vi "Host_Model_Updating.vi"(11 "Setup Parameters and Controls":T3={"Modeling Parameters input controls"={"beam_length"=0.3525, "youngs_modulus"=209500000000.0, "torsion_spring"=0.0, "beam_height"=0.00635, "beam_width"=0.0508, "beam_density"=7900.0, "number_of_FEA_nodes"=40, "accelerometer_mass"=0.055}, "Mockbear input controls"={"Dataset"="test7", "Resample Method"=enum."Auto Resample"}, "Simulation Parameters input controls"={"Eigensolver "=enum."LEMP", "Models Forcasted"=5, "Max Roller Velocity"=3.32, "Max Roller Position Percent"=0.43, "Min Roller Position Percent"=0.155}, "Program Controls"={"Frequency KF"=TRUE, "Pinned State KF"=FALSE, "FFT Bounding"=FALSE, "Filter Constants Frequency"={"Measurement Variance"=0.4, "State Variance"=0.01, "Threshold"=1000000000.0}, "Filter Constants Position"={"Measurement Variance"=0.4, "State Variance"=0.9, "Threshold"=1000000000.0}, "Moving Window Size"=10, "Time Series buffer"=10000.0, "Record Time Series Data"=FALSE, "Record Moving Window Data"=FALSE, "Record Online Error Metrics "=TRUE, "Record Statistics"=TRUE}}) -> ()   [LabVIEW 2021]
uses:
  Model_Updating_Classes/DROPBEAR_Model_Updating/DROPBEAR_Model_Updating.lvclass
panel:
  in  "Tab Control":enum32{"Time Series", "Statistics", "Controls"}(tab)
  out "Frequency":dynamicdata(graph)
  out "Meter":dynamicdata(graph)
  out "Nodal":dynamicdata(graph)
  out "DAQ Time cost":T1
  out "FFT Time cost":T1
  out "FEA Time cost":T1
  out "FFT KF Time cost":T1
  out "Sampling Time cost":T1
  out "State KF Time cost":T1
  out "Cycle Time cost":T1
  out "StatisticsTime cost":T1
  out "Signal Quality Stats Frequency":T2
  out "Signal Quality Stats Position":T2
  out "Average Cycle Time (ms)":dbl
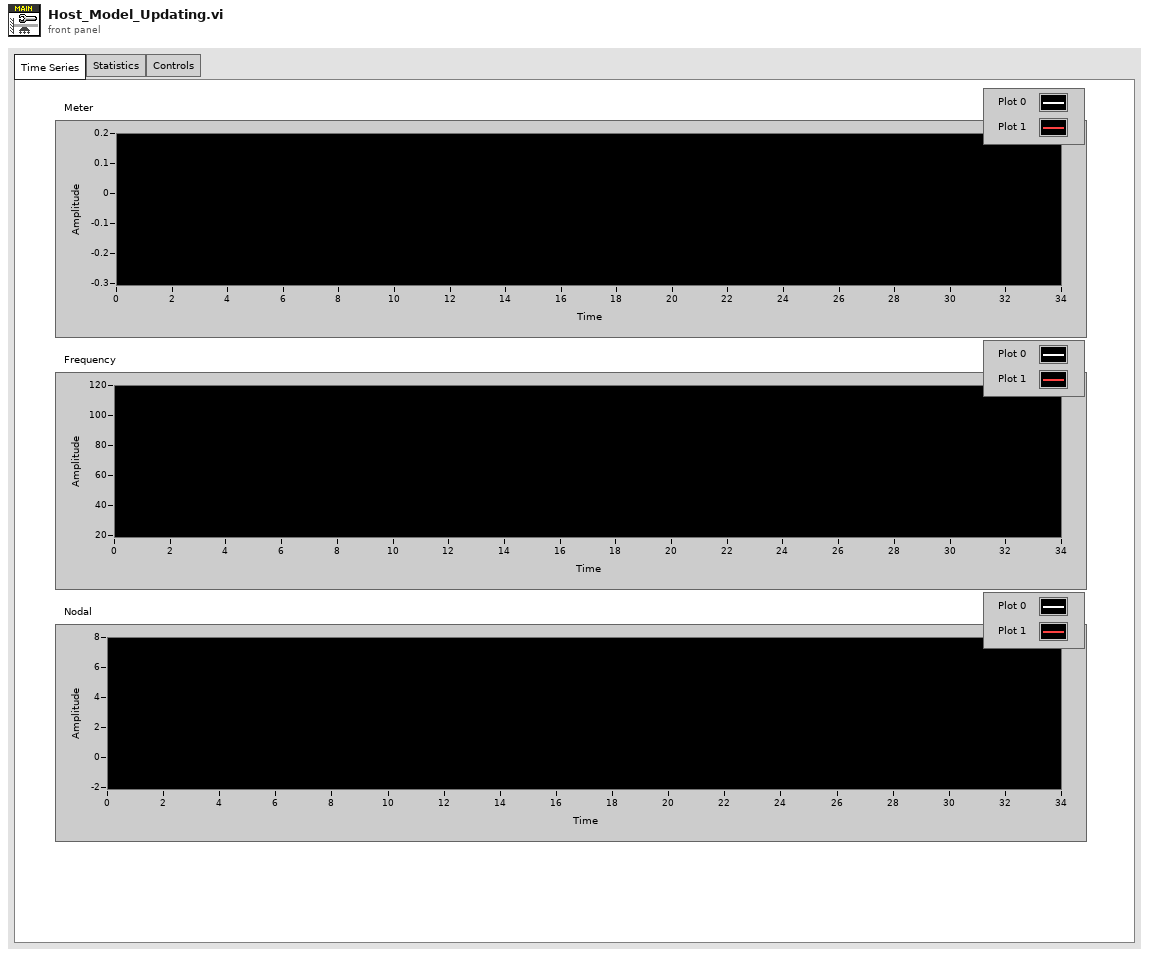
[diagram p1: front panel]
types:
  T1 = cluster{"Cumulative_mean":dbl, "Cumulative_mean_square ":dbl, "Cumulative_variance":dbl, "Max":dbl, "Min":dbl, "Number_of_samples":i32}
  T2 = cluster{"SNR":dbl, "TRAC":dbl, "Cumulative_mean":dbl, "Cumulative_mean_square ":dbl, "Cumulative_variance":dbl, "Max":dbl, "Min":dbl, "Number_of_samples":i32}
  T3 = cluster{"Modeling Parameters input controls":cluster{"beam_length":dbl, "youngs_modulus":dbl, "torsion_spring":dbl, "beam_height":dbl, "beam_width":dbl, "beam_density":dbl, "number_of_FEA_nodes":i32, "accelerometer_mass":dbl}, "Mockbear input controls":cluster{"Dataset":string, "Resample Method":enum16{"Recorded", "Auto Resample", "Custom Resample"}}, "Simulation Parameters input controls":cluster{"Eigensolver ":enum16{"LabVIEW Cholesky", "LabVIEW General", "LabVIEW Inverse", "LEMP"}, "Models Forcasted":i32, "Max Roller Velocity":dbl, "Max Roller Position Percent":dbl, "Min Roller Position Percent":dbl}, "Program Controls":cluster{"Frequency KF":bool, "Pinned State KF":bool, "FFT Bounding":bool, "Filter Constants Frequency":cluster{"Measurement Variance":dbl, "State Variance":dbl, "Threshold":dbl}, "Filter Constants Position":cluster{"Measurement Variance":dbl, "State Variance":dbl, "Threshold":dbl}, "Moving Window Size":i32, "Time Series buffer":dbl, "Record Time Series Data":bool, "Record Moving Window Data":bool, "Record Online Error Metrics ":bool, "Record Statistics":bool}}
  T4 = cluster{"Signal Quality Stats Frequency":cluster{"SNR":dbl, "TRAC":dbl, "Cumulative_mean":dbl, "Cumulative_mean_square ":dbl, "Cumulative_variance":dbl, "Max":dbl, "Min":dbl, "Number_of_samples":i32}, "Signal Quality Stats Position":cluster{"SNR":dbl, "TRAC":dbl, "Cumulative_mean":dbl, "Cumulative_mean_square ":dbl, "Cumulative_variance":dbl, "Max":dbl, "Min":dbl, "Number_of_samples":i32}}
  T5 = cluster{"DAQ Time cost":cluster{"Cumulative_mean":dbl, "Cumulative_mean_square ":dbl, "Cumulative_variance":dbl, "Max":dbl, "Min":dbl, "Number_of_samples":i32}, "FFT Time cost":cluster{"Cumulative_mean":dbl, "Cumulative_mean_square ":dbl, "Cumulative_variance":dbl, "Max":dbl, "Min":dbl, "Number_of_samples":i32}, "FFT KF Time cost":cluster{"Cumulative_mean":dbl, "Cumulative_mean_square ":dbl, "Cumulative_variance":dbl, "Max":dbl, "Min":dbl, "Number_of_samples":i32}, "Sampling Time cost":cluster{"Cumulative_mean":dbl, "Cumulative_mean_square ":dbl, "Cumulative_variance":dbl, "Max":dbl, "Min":dbl, "Number_of_samples":i32}, "FEA Time cost":cluster{"Cumulative_mean":dbl, "Cumulative_mean_square ":dbl, "Cumulative_variance":dbl, "Max":dbl, "Min":dbl, "Number_of_samples":i32}, "State KF Time cost":cluster{"Cumulative_mean":dbl, "Cumulative_mean_square ":dbl, "Cumulative_variance":dbl, "Max":dbl, "Min":dbl, "Number_of_samples":i32}, "Cycle Time cost":cluster{"Cumulative_mean":dbl, "Cumulative_mean_square ":dbl, "Cumulative_variance":dbl, "Max":dbl, "Min":dbl, "Number_of_samples":i32}, "StatisticsTime cost":cluster{"Cumulative_mean":dbl, "Cumulative_mean_square ":dbl, "Cumulative_variance":dbl, "Max":dbl, "Min":dbl, "Number_of_samples":i32}}
  T6 = cluster{"Frequency":dynamicdata, "Meters":dynamicdata, "Nodal":dynamicdata}
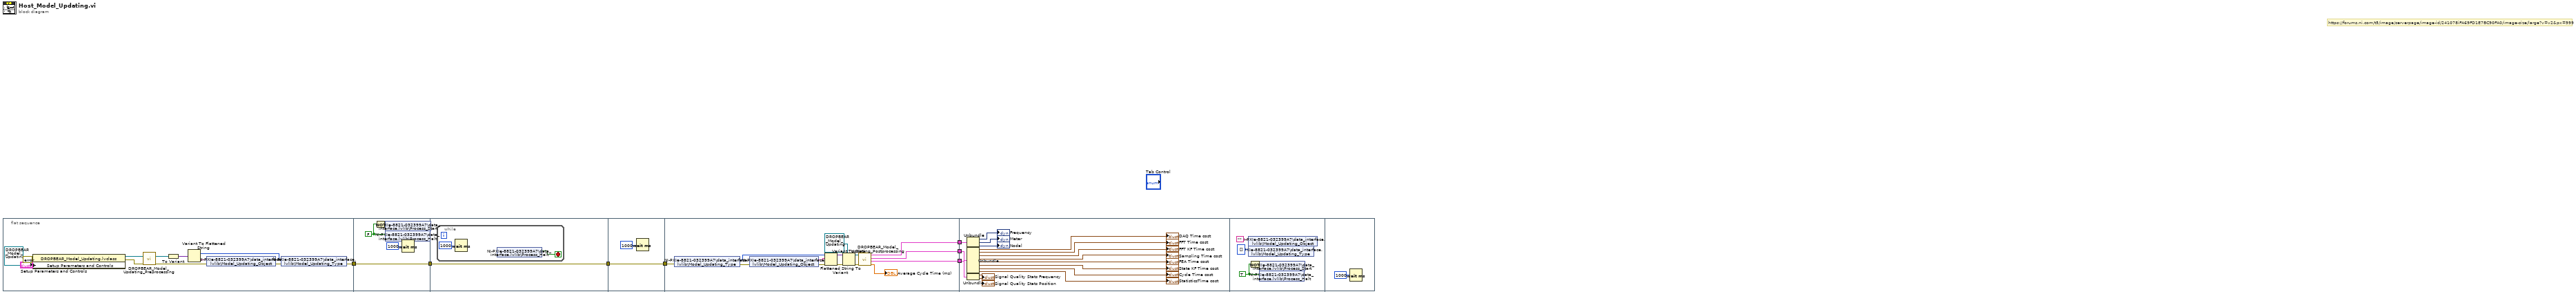
[diagram p0: block diagram]
diagram:
  # "https://forums.ni.com/t5/image/serverpage/image-id/241078iFA69FD1E7BC90FA0/image-size/large?v=v2&px=999"
  n1 = flat-sequence {
    tunnel: [w14] -> w4
    tunnel: w4 -> [w20]
    tunnel: [w20] -> w1
    tunnel: [w24] -> w3
    tunnel: w1 -> [w24]
    tunnel: w3 -> [w27]
    tunnel: [w27] -> w2
    tunnel: [w31] -> w7
    tunnel: [w30] -> w6
    tunnel: [w29] -> w5
    tunnel: w2 -> [w34]
    tunnel: w5 -> [w58]
    tunnel: w6 -> [w55]
    tunnel: w7 -> [w46]
    frame #0 {
      n2 = property class="DROPBEAR_Model_Updating.lvclass"(reference=refnum<class "DROPBEAR_Model_Updating.lvclass"> refnum ("DROPBEAR_Model_Updating.lvclass"), error in=errorcluster {"status"=FALSE, "code"=0, "source"=""} ("error in (no error)"), "Setup Parameters and Controls"="Setup Parameters and Controls") -> (reference out=w13:refnum<class "DROPBEAR_Model_Updating.lvclass">, error out=w9:errorcluster)
      n3 = call-dynamic "DROPBEAR_Model_Updating_Preprocessing.vi"("error in (no error)"=w9, "DROPBEAR_Model_Updating in"=w13) -> ("error out"=w18:errorcluster, "DROPBEAR_Model_Updating out"=w19:refnum<class "DROPBEAR_Model_Updating.lvclass">)  [unwired: 8 in]
      n4 = To Variant(anything=w19) -> (Variant=w17:variant)
      n5 = Variant To Flattened String(Variant=w17) -> (data string=w16:string, 1:w8:i16[])
      n6 = shared-variable "NI-PXIe-8821-032399A7\\data_interface.lvlib\\Model_Updating_Object"(w16, error in=w18) -> (error out=w15:errorcluster)
      n7 = shared-variable "NI-PXIe-8821-032399A7\\data_interface.lvlib\\Model_Updating_Type"(w8, error in=w15) -> (error out=w14:errorcluster)
    }
    frame #1 {
      w21 = FALSE ("Process_Halt")
      n8 = Not(x=w21) -> (.not. x?=w22:bool)
      n9 = shared-variable "NI-PXIe-8821-032399A7\\data_interface.lvlib\\Process_Start"(w22) -> ()  [unwired: 1 in, 1 out]
      n10 = shared-variable "NI-PXIe-8821-032399A7\\data_interface.lvlib\\Process_Halt"(w21) -> ()  [unwired: 1 in, 1 out]
      n11 = Wait (ms)(milliseconds to wait=u32 1000) -> ()  [unwired: 1 out]
    }
    frame #2 {
      n12 = while {
        stop <- w26 stop-if-true
        n13 = Wait (ms)(milliseconds to wait=u32 1000) -> ()  [unwired: 1 out]
        n14 = shared-variable "NI-PXIe-8821-032399A7\\data_interface.lvlib\\Process_Halt"() -> (w26:bool)  [unwired: 1 in, 1 out]
      }
    }
    frame #3 {
      n15 = Wait (ms)(milliseconds to wait=u32 1000) -> ()  [unwired: 1 out]
    }
    frame #4 {
      n16 = shared-variable "NI-PXIe-8821-032399A7\\data_interface.lvlib\\Model_Updating_Type"(error in=w34) -> (w38:i16[], error out=w41:errorcluster)
      n17 = shared-variable "NI-PXIe-8821-032399A7\\data_interface.lvlib\\Model_Updating_Object"(error in=w41) -> (w39:string, error out=w40:errorcluster)
      n18 = Flattened String To Variant(4:w40, 6:w39, 7:w38) -> (0:w35:errorcluster, 3:w36:variant)
      n19 = Variant To Data(error in=w35, type=refnum<class "DROPBEAR_Model_Updating.lvclass"> refnum ("DROPBEAR_Model_Updating.lvclass"), Variant=w36) -> (data=w33:refnum<class "DROPBEAR_Model_Updating.lvclass">, error out=w32:errorcluster)
      n20 = call "DROPBEAR_Model_Updating_Postprocessing.vi"("error in (no error)"=w32, "DROPBEAR_Model_Updating in"=w33) -> ("Cycle time (ms)"=→"Average Cycle Time (ms)":dbl, "Signal Quality"=w29:T4, "Timing stats"=w30:T5, "Plots"=w31:T6)  [unwired: 6 in]
    }
    frame #5 {
      n21 = Unbundle(w46) -> ("Frequency"=→"Frequency":dynamicdata, "Meters"=→"Meter":dynamicdata, "Nodal"=→"Nodal":dynamicdata)
      n22 = Unbundle(w55) -> ("DAQ Time cost"=→"DAQ Time cost":T1, "FFT Time cost"=→"FFT Time cost":T1, "FFT KF Time cost"=→"FFT KF Time cost":T1, "Sampling Time cost"=→"Sampling Time cost":T1, "FEA Time cost"=→"FEA Time cost":T1, "State KF Time cost"=→"State KF Time cost":T1, "Cycle Time cost"=→"Cycle Time cost":T1, "StatisticsTime cost"=→"StatisticsTime cost":T1)
      n23 = Unbundle(w58) -> ("Signal Quality Stats Frequency"=→"Signal Quality Stats Frequency":T2, "Signal Quality Stats Position"=→"Signal Quality Stats Position":T2)
    }
    frame #6 {
      w60 = TRUE ("Process_Halt")
      n24 = shared-variable "NI-PXIe-8821-032399A7\\data_interface.lvlib\\Model_Updating_Object"("") -> ()  [unwired: 1 in, 1 out]
      n25 = shared-variable "NI-PXIe-8821-032399A7\\data_interface.lvlib\\Model_Updating_Type"(i16[] [] ("Model_Updating_Type")) -> ()  [unwired: 1 in, 1 out]
      n26 = Not(x=w60) -> (.not. x?=w59:bool)
      n27 = shared-variable "NI-PXIe-8821-032399A7\\data_interface.lvlib\\Process_Start"(w59) -> ()  [unwired: 1 in, 1 out]
      n28 = shared-variable "NI-PXIe-8821-032399A7\\data_interface.lvlib\\Process_Halt"(w60) -> ()  [unwired: 1 in, 1 out]
    }
    frame #7 {
      n29 = Wait (ms)(milliseconds to wait=u32 1000) -> ()  [unwired: 1 out]
    }
  }
